vi "IRCheck_Main_Robot_Control.vi"() -> ()   [LabVIEW 2014]
panel:
  in  "Tab Control":T1(tab)
  out "Raw Volts":dbl
  out "Center_JR":dbl(slide) scale=0.0..3.0
  out "Pot":dbl(slide) min=0.0 max=5.0 step=0.25 scale=0.0..5.0
  in  "Motor Direction":bool
  in  "1) SET Start Position of Head":dbl
  out "Sensor Head Position":dbl
  out "?":dbl(knob) scale=-800.0..800.0
  out "Stop Engaged":bool
  in  "?":bool
  out "Blinky Light":bool
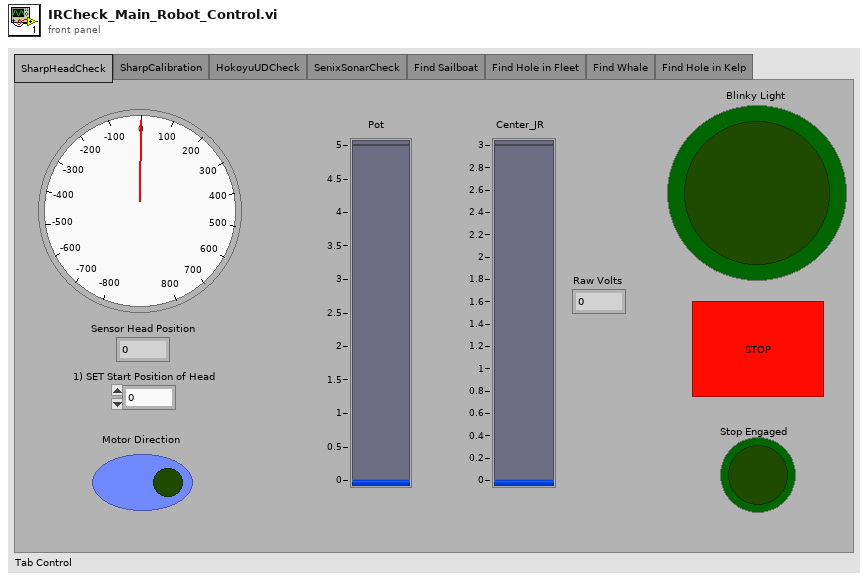
[diagram p1: front panel]
types:
  T1 = enum32{"SharpHeadCheck", "SharpCalibration", "HokoyuUDCheck", "SenixSonarCheck", "Find Sailboat", "Find Hole in Fleet", "Find Whale", "Find Hole in Kelp"}
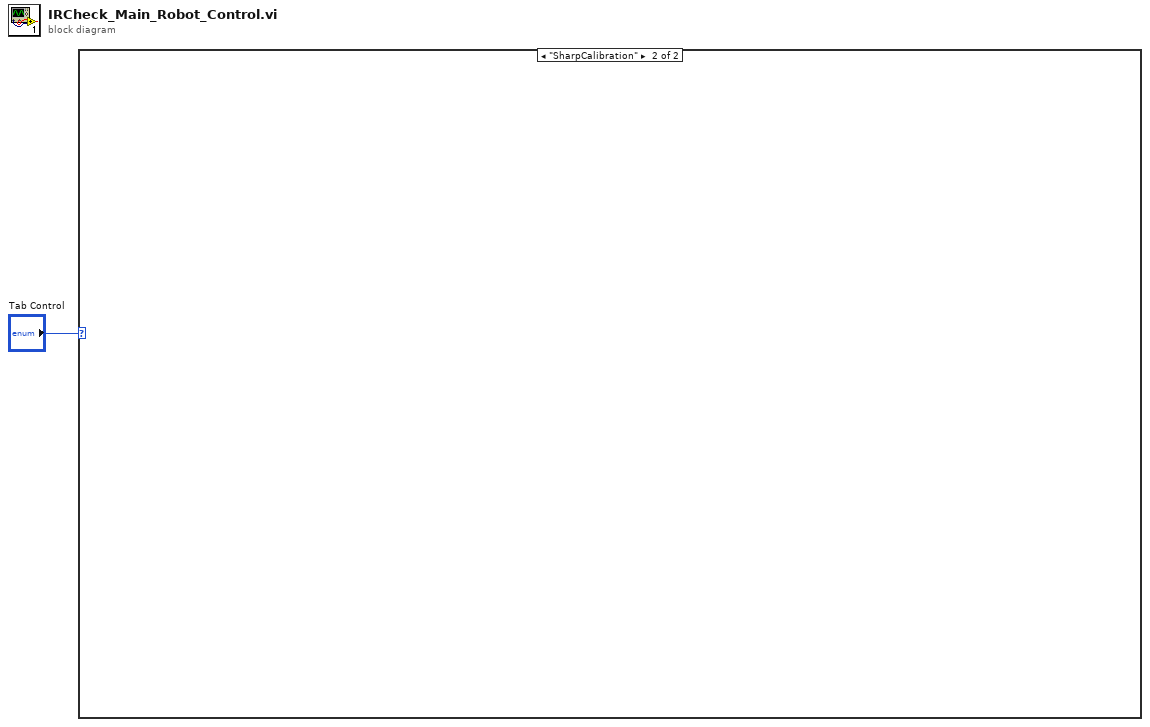
[diagram p0: block diagram]
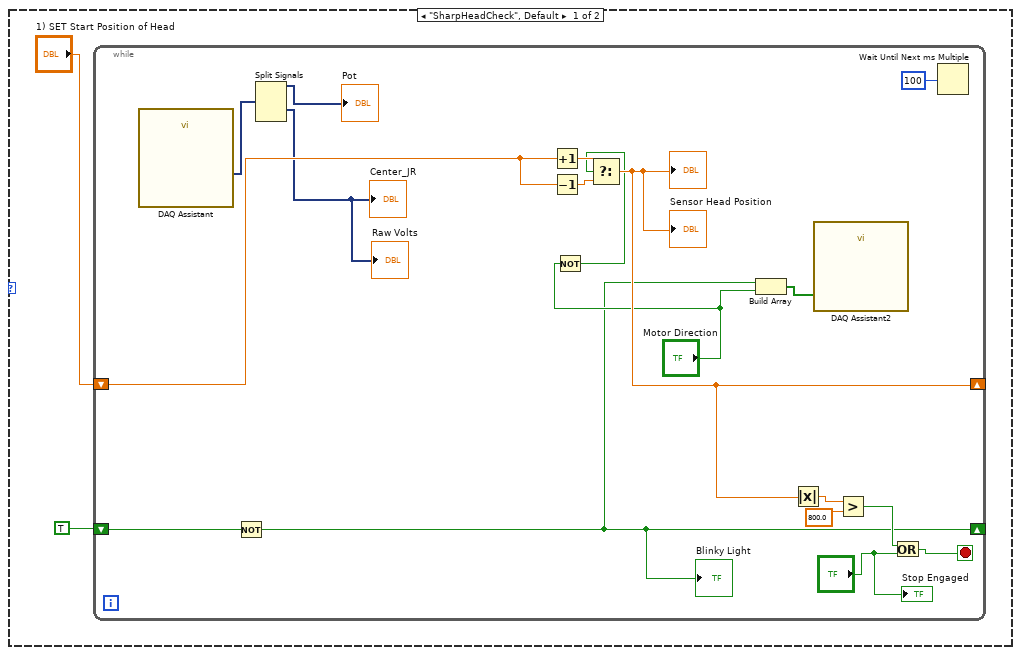
[diagram p2: hidden frame]
diagram:
  n1 = case shown="\"SharpCalibration\"" "Tab Control" {
    frame "SharpHeadCheck", Default {
      n2 = while {
        shift-right: [w12] -> _
        shift-left: "1) SET Start Position of Head" -> [w14]
        shift-right: [w4] -> _
        shift-left: TRUE -> [w5]
        stop <- w21 stop-if-true
        n3 = call "DAQ Assistant"() -> ("data"=w9:dynamicdata)  [unwired: 17 in, 2 out]
        n4 = Not(x=w5) -> (.not. x?=w4:bool)
        "Blinky Light" <- w4
        n5 = Split Signals(w9) -> (→"Pot":dynamicdata, →"Center_JR" →"Raw Volts":dynamicdata)  [unwired: 5 in, 3 out]
        n6 = Increment(x=w14) -> (x+1=w16:dbl)
        n7 = Decrement(x=w14) -> (x-1=w15:dbl)
        n8 = Not(x="Motor Direction") -> (.not. x?=w11:bool)
        n9 = Select(t=w16, s=w11, f=w15) -> (s? t:f=w12:dbl)
        "Sensor Head Position" <- w12
        "?" <- w12
        n10 = Build Array(w4, "Motor Direction") -> (w6:bool[])
        n11 = Absolute Value(x=w12) -> (abs(x)=w17:dbl)
        n12 = call "DAQ Assistant2"("data"=w6) -> ()  [unwired: 17 in, 2 out]
        n13 = Greater?(x=w17, y=800.0) -> (0:w19:bool)
        n14 = Or(x=w19, y="?") -> (x .or. y?=w21:bool)
        n15 = Wait Until Next ms Multiple(millisecond multiple=100) -> ()  [unwired: 1 out]
        "Stop Engaged" <- "?"
      }
    }
    frame "SharpCalibration" {
    }
  }
